vi "Register Channel.vi"(8 "error in (no error)":errorcluster, 10 "Channel":refnum<class "CIFChannels.lvclass">, 11 "CIFCorePlugin in":refnum<class "CIFCorePlugin.lvclass">) -> (0 "error out":errorcluster, 3 "CIFCorePlugin out":refnum<class "CIFCorePlugin.lvclass">)   [LabVIEW 2021, in "CIFCorePlugin.lvclass"]
uses:
  CIFCorePlugin.lvclass
  <vilib>/CIF Foundation/CIF Channels Core/CIFChannels/CIFChannels.lvclass
  CIFCorePlugin.lvclass/CIFCorePlugin.ctl
  <vilib>/CIF Foundation/CIF Channels Core/CIFChannels/CIFChannels.lvclass/CIFChannels.ctl
  Channels/CIFChannelMng/CIFChannelMng.lvclass/CIFChannelMng.ctl
  <vilib>/CIF Foundation/CIF Channels Core/ChannelCommon/Utilities/Add Error.vi
  <vilib>/CIF Foundation/CIF Channels Core/CIFChannels/Accessors/Read Name.vi
  <vilib>/CIF Foundation/CIF Channels Core/CIFChannels/Accessors/Read Custom Config Data.vi
  <vilib>/CIF Foundation/CIF Channels Core/CIFChannels/Accessors/Read Type.vi
  <vilib>/CIF Foundation/CIF Channels Core/CIFChannels/Accessors/Read Pattern.vi
  <vilib>/CIF Foundation/CIF Channels Core/CIFChannels/Accessors/Read Direction.vi
  <vilib>/CIF Foundation/CIF Channels Core/CIFChannels/Accessors/Read Channel State.vi
  <vilib>/CIF Foundation/CIF Utilities/Errors/Append Error Location.vi
  Channels/CIFChannelMng/CIFChannelMng.lvclass
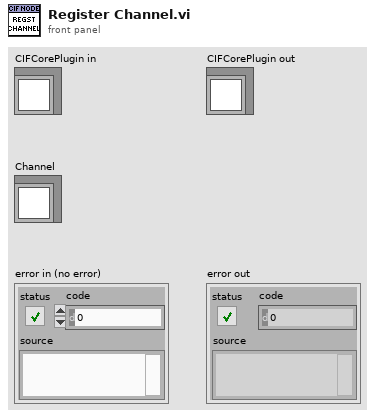
[diagram p1: front panel]
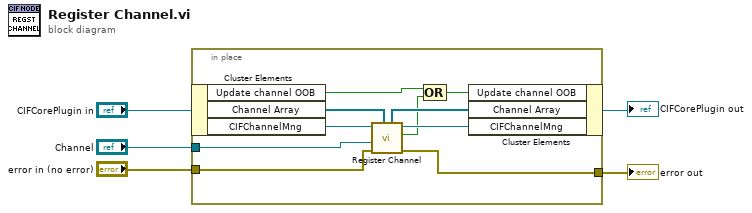
[diagram p0: block diagram]
diagram:
  n1 = in-place {
    in-place-border: "error in (no error)" -> [w11]
    in-place-border: "Channel" -> [w10]
    in-place-border: [w9] -> w2
    n2 = in-place-cluster #1("CIFCorePlugin in") -> ("Update channel OOB"=w6:bool, "Channel Array"=w13:refnum<class "CIFChannels.lvclass">[], "CIFChannelMng"=w15:refnum<class "CIFChannelMng.lvclass">)
    n3 = call "Register Channel.vi"("Channel Array in"=w13, "error in (no error)"=w11, "Channel"=w10, "CIFChannelMng in"=w15) -> ("error out"=w9:errorcluster, "Update Channel OOB"=w8:bool, "CIFChannelMng out"=w14:refnum<class "CIFChannelMng.lvclass">, "Channel Array out"=w12:refnum<class "CIFChannels.lvclass">[])  [unwired: 4 in]
    n4 = Compound Arithmetic op=OR(w6, w8) -> (w7:bool)
    n5 = in-place-cluster #1("Update channel OOB"=w7, "Channel Array"=w12, "CIFChannelMng"=w14) -> (→"CIFCorePlugin out":refnum<class "CIFCorePlugin.lvclass">)
  }
  "error out" <- w2
